vi "Curtin1_ReadSaveTemplate.vi"(6 "Task":enum16{"Save", "Read", "List"}(ring), 9 "Template":string="favorites.txt", 11 "Settings":T1={"Name of test"="ScratchPad", "Date"=timestamp(0 s since 1904-01-01), "Location"="Home", "Template"="Simple", "Soundcard"="OCTA-CAPTURE", "resolution"=32, "Sampling rate"=48000, "Ch1 Gain "=25.0, "Ch2 Gain"=10.0, "Sample time (s)"=0.3, "Pre-trigger (s)"=0.001, "Hammer Threshold"=10.0, "Positions"=12, "Taps/Position"=5, "Set Names"="H,V", "Freq resolution"=1.0, "Hammer cutoff"=0.025, "Mic cutoff"=0.25, "Double bounce "=10.0, "Hammer Cal"=10.0, "dB Offset"=0.0, "Accel Cal"=10.0, "Vibrometer Cal"=0.0, "Mic Cal"=0.0, "Output"=2, "Voltage Cal"=1.0, "Vibrometer Port"="ASRL27::INSTR", "Range"=4, "High Pass"=2, "Bandwidth"=4, "X Range"=[], "Y Range"=[], "dB Spread"=0.0, "Trigger"=0, "Ch_1"=25, "Ch_2"=25, "flip?"=FALSE, "60Hz"=FALSE, "Time offset"=0.0, "Piezo Cal"=1.0, "Default Notes"=""} {"Ch_2" min=1 step=1; "Ch_1" min=1 max=100 step=1; "Trigger" items=["Hammer (force)", "Self-tap", "Spacebar"]; "Bandwidth" items=["1 kHz"=1, "5 kHz"=5, "10 kHz"=10, "25 kHz"=25, "50 kHz"=50, "100 kHz"=100]; "High Pass" items=["Off", "13 Hz", "104 Hz"]; "Range" items=["10 mm/s"=1, "20 mm/s"=2, "50 mm/s"=5, "100 mm/s"=10, "200 mm/s"=20, "500 mm/s"=50, "1 m/s"=100, "2 m/s"=200]; "Output" items=["Accelerometer", "Speed (from acceleration)", "Microphone", "Vibrometer", "Piezo"]; "Voltage Cal" format="%#_13g"; "Ch2 Gain" format="%#_13g"; "Ch1 Gain" format="%#_13g"; "Double bounce" min=0.0; "Mic cutoff" min=0.0 format="%#_4g"; "Hammer cutoff" min=0.0 format="%#_4g"; "Freq resolution" min=0.0; "Pre-trigger (s)" format="%#_13g"; "Date" format="%<%H:%M\n%d/%m/%y>T"; "resolution" items=["16 bit"=16, "24 bit"=24, "32 bit"=32]; "Sampling rate" items=["22050 samp/s"=22050, "44100 samp/s"=44100, "48000 samp/s"=48000]}) -> (0 "error out":errorcluster, 1 "String":string, 2 "List":string[](array[string]), 3 "Settings out":T1={"Name of test"="", "Date"=timestamp(0 s since 1904-01-01), "Location"="", "Template"="", "Soundcard"="", "resolution"=32, "Sampling rate"=48000, "Ch1 Gain "=25.0, "Ch2 Gain"=10.0, "Sample time (s)"=0.3, "Pre-trigger (s)"=0.01, "Hammer Threshold"=10.0, "Positions"=12, "Taps/Position"=5, "Set Names"="", "Freq resolution"=10.0, "Hammer cutoff"=0.0, "Mic cutoff"=0.0, "Double bounce "=0.0, "Hammer Cal"=10.0, "dB Offset"=0.0, "Accel Cal"=10.0, "Vibrometer Cal"=0.0, "Mic Cal"=0.0, "Output"=2, "Voltage Cal"=1.0, "Vibrometer Port"="ASRL27::INSTR", "Range"=4, "High Pass"=2, "Bandwidth"=4, "X Range"=[], "Y Range"=[], "dB Spread"=0.0, "Trigger"=0, "Ch_1"=25, "Ch_2"=25, "flip?"=FALSE, "60Hz"=FALSE, "Time offset"=0.0, "Piezo Cal"=1.0, "Default Notes"=""} {"Ch_2" min=1 step=1; "Ch_1" min=1 max=100 step=1; "Trigger" items=["Hammer (force)", "Self-tap", "Spacebar"]; "Bandwidth" items=["1 kHz"=1, "5 kHz"=5, "10 kHz"=10, "25 kHz"=25, "50 kHz"=50, "100 kHz"=100]; "High Pass" items=["Off", "13 Hz", "104 Hz"]; "Range" items=["10 mm/s"=1, "20 mm/s"=2, "50 mm/s"=5, "100 mm/s"=10, "200 mm/s"=20, "500 mm/s"=50, "1 m/s"=100, "2 m/s"=200]; "Output" items=["Accelerometer", "Speed (from acceleration)", "Microphone", "Vibrometer", "Piezo"]; "Voltage Cal" format="%#_13g"; "Ch2 Gain" format="%#_13g"; "Ch1 Gain" format="%#_13g"; "Double bounce" min=0.0; "Mic cutoff" min=0.0 format="%#_4g"; "Hammer cutoff" min=0.0 format="%#_4g"; "Freq resolution" min=0.0; "Pre-trigger (s)" format="%#_13g"; "Date" format="%<%H:%M\n%d/%m/%y>T"; "resolution" items=["16 bit"=16, "24 bit"=24, "32 bit"=32]; "Sampling rate" items=["22050 samp/s"=22050, "44100 samp/s"=44100, "48000 samp/s"=48000]})   [LabVIEW 2022 SP3]
uses:
  PreferencesControl.ctl
  Mic/Mic_Global.vi
panel:
  # "Hz"
  # "dB"
  # "dB"
  # "sec"
  # "sec"
  # "mV/Pa"
  # "mV/m/s2"
  # "mV/mm/s"
  # "V/N"
  # "sec"
  # "sec"
  # "mV/N"
  # "a.u."
  # "a.u."
  # "sec"
  # "Hz"
  # "dB"
  # "dB"
  # "sec"
  # "sec"
  # "mV/Pa"
  # "mV/m/s2"
  # "mV/mm/s"
  # "V/N"
  # "sec"
  # "sec"
  # "mV/N"
  # "a.u."
  # "a.u."
  # "sec"
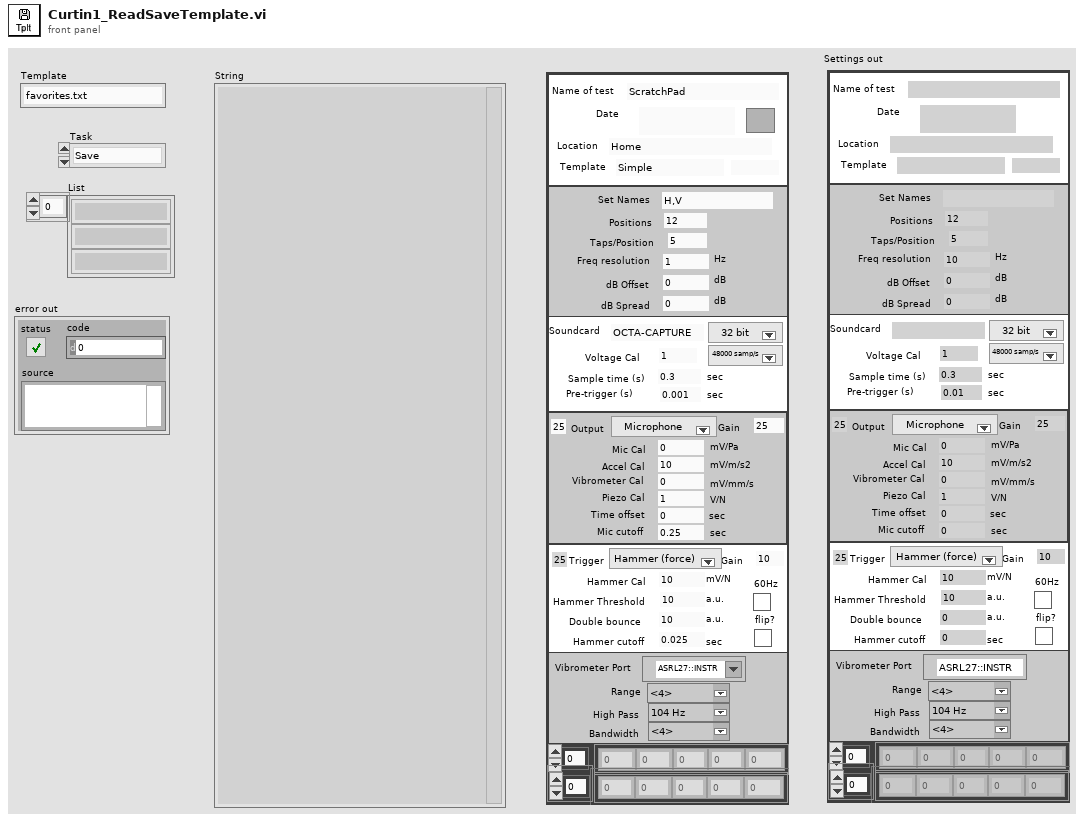
[diagram p1: front panel]
types:
  T1 = typedef "PreferencesControl.ctl" = cluster{"Name of test":string, "Date":timestamp, "Location":string, "Template":string, "Soundcard":string, "resolution":u16, "Sampling rate":u16, "Ch1 Gain ":dbl, "Ch2 Gain":dbl, "Sample time (s)":dbl, "Pre-trigger (s)":dbl, "Hammer Threshold":dbl, "Positions":i16, "Taps/Position":i16, "Set Names":string, "Freq resolution":dbl, "Hammer cutoff":dbl, "Mic cutoff":dbl, "Double bounce ":dbl, "Hammer Cal":dbl, "dB Offset":dbl, "Accel Cal":dbl, "Vibrometer Cal":dbl, "Mic Cal":dbl, "Output":u16, "Voltage Cal":dbl, "Vibrometer Port":refnum<visa-resource-name>, "Range":u16, "High Pass":u16, "Bandwidth":u16, "X Range":cluster{"Minimum":dbl, "Maximum":dbl, "Increment":dbl, "Minor Increment":dbl, "Start":dbl}[], "Y Range":cluster{"Minimum":dbl, "Maximum":dbl, "Increment":dbl, "Minor Increment":dbl, "Start":dbl}[], "dB Spread":dbl, "Trigger":u16, "Ch_1":u8, "Ch_2":u8, "flip?":bool, "60Hz":bool, "Time offset":dbl, "Piezo Cal":dbl, "Default Notes":string}
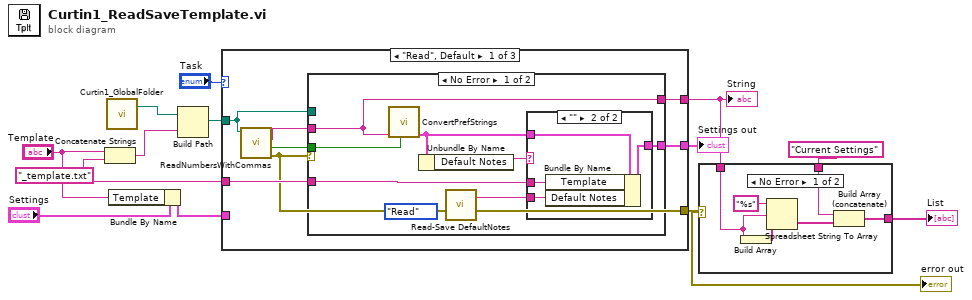
[diagram p0: block diagram]
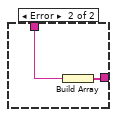
[diagram p2: hidden frame]
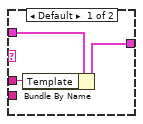
[diagram p3: hidden frame]
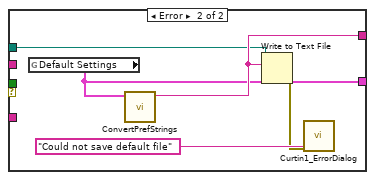
[diagram p4: hidden frame]
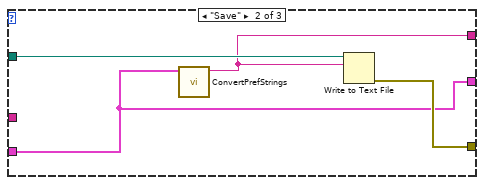
[diagram p5: hidden frame]
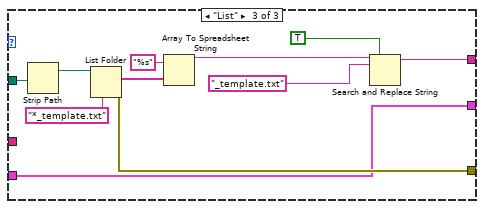
[diagram p6: hidden frame]
diagram:
  n1 = Concatenate Strings("Template", "_template.txt" ("string")) -> (w3:string)
  n2 = call "Curtin1_GlobalFolder.vi"() -> ("LabVIEW Data Path"=w5:path)  [unwired: 1 in, 1 out]
  n3 = Bundle By Name(cluster="Settings", "Template"="Template") -> (w2:T1)
  n4 = Build Path(base path=w5, name or relative path=w3) -> (appended path=w13:path)
  n5 = case shown="\"Read\", Default" "Task" {
    tunnel: w13 -> [w17 w44 w55]
    tunnel: [w15 w43 w46] -> w7
    tunnel: [w20 w42 w50] -> w9
    tunnel: [w19 w41 w45] -> w6
    tunnel: w2 -> [_ w41 w45]
    tunnel: "Template" -> [w18 _ _]
    frame "Read", Default {
      n6 = call "ReadNumbersWithCommas.vi"("file (use dialog)"=w17) -> ("error out"=w15:errorcluster, "comma?"=w14:bool, "text"=w16:string)  [unwired: 7 in, 1 out]
      n7 = case shown="No Error" w15 {
        tunnel: w16 -> [w28 _]
        tunnel: [w28 w40] -> w20
        tunnel: [w26 w39] -> w19
        tunnel: w17 -> [_ w38]
        tunnel: w18 -> [w27 _]
        tunnel: w14 -> [w25 _]
        frame No Error {
          n8 = call "ConvertPrefStrings.vi"("Comma?"=w25, "String In"=w28) -> ("Settings"=w24:T1)  [unwired: 8 in, 1 out]
          n9 = Unbundle By Name(w24) -> ("Default Notes"=w23:string)
          n10 = call "Read-Save DefaultNotes.vi"("Task"=enum16{"Save", "Read"}."Read") -> ("Notes Out"=w22:string)  [unwired: 9 in, 1 out]
          n11 = case shown="\"\"" w23 {
            tunnel: w27 -> [w31 w35]
            tunnel: [w30 w33] -> w26
            tunnel: w24 -> [w29 w34]
            tunnel: w22 -> [_ w32]
            frame Default {
              n12 = Bundle By Name(cluster=w29, "Template"=w31) -> (w30:T1)
            }
            frame "" {
              n13 = Bundle By Name(cluster=w34, "Template"=w35, "Default Notes"=w32) -> (w33:T1)
            }
          }
        }
        frame Error {
          n14 = global read "Mic_Global.vi" "Default Settings"() -> (w39:T1)
          n15 = call "ConvertPrefStrings.vi"("Settings"=w39) -> ("String Out"=w40:string)  [unwired: 9 in, 1 out]
          n16 = Write to Text File(file (use dialog)=w38, text=w40) -> (error out=w36:errorcluster)  [unwired: 2 in, 2 out]
          n17 = call "Curtin1_ErrorDialog.vi"("error in (no error)"=w36, "String"="Could not save default file") -> ()  [unwired: 9 in, 1 out]
        }
      }
    }
    frame "Save" {
      n18 = call "ConvertPrefStrings.vi"("Settings"=w41) -> ("String Out"=w42:string)  [unwired: 9 in, 1 out]
      n19 = Write to Text File(file (use dialog)=w44, text=w42) -> (error out=w43:errorcluster)  [unwired: 2 in, 2 out]
    }
    frame "List" {
      n20 = Strip Path(path=w55) -> (stripped path=w54:path)  [unwired: 1 out]
      n21 = List Folder(path=w54, pattern="*_template.txt") -> (filenames=w52:string[], error out=w46:errorcluster)  [unwired: 2 in, 2 out]
      n22 = Array To Spreadsheet String(array=w52, 3:"%s" ("format string")) -> (spreadsheet string=w49:string)  [unwired: 1 in]
      n23 = Search and Replace String(replace all?=TRUE ("replace all? (F)"), input string=w49, search string="_template.txt") -> (result string=w50:string)  [unwired: 5 in, 3 out]
    }
  }
  "String" <- w9
  "Settings out" <- w6
  "error out" <- w7
  n24 = case shown="No Error" w7 {
    tunnel: "Current Settings" ("String") -> [w58 w63]
    tunnel: w9 -> [w57 _]
    tunnel: [w56 w62] -> w8
    frame No Error {
      n25 = Build Array(w57) -> (w61:string[])
      n26 = Spreadsheet String To Array(format string="%s", spreadsheet string=w57, array type (2D Dbl)=w61) -> (array=w59:string[])  [unwired: 1 in]
      n27 = Build Array (concatenate)(w58, w59) -> (w56:string[])
    }
    frame Error {
      n28 = Build Array(w63) -> (w62:string[])
    }
  }
  "List" <- w8
